vi "Record Defaults in Log File.vi"(6 "Application":refnum<class "Application.lvclass">, 7 "Position":u32, 8 "error in (no error)":errorcluster, 11 "Parameter Loader in":refnum<class "Parameter Loader.lvclass">) -> (0 "error out":errorcluster)   [LabVIEW 2015, in "Load Defaults.lvclass"]
uses:
  Load Defaults.lvclass
  Classes/Parameter Loader/Class/Parameter Loader.lvclass
  Classes/Application/Class/Application.lvclass
  <vilib>/Cree, Inc/Cree Test Framework/Core Launcher/Core Manager Methods -- Enum.ctl
  <vilib>/Cree, Inc/Cree Test Framework/Core Launcher/Core Launcher.lvlib
  <vilib>/Cree, Inc/Cree Test Framework/Classes/Data/Data Repo/Class/Data Repo.lvclass
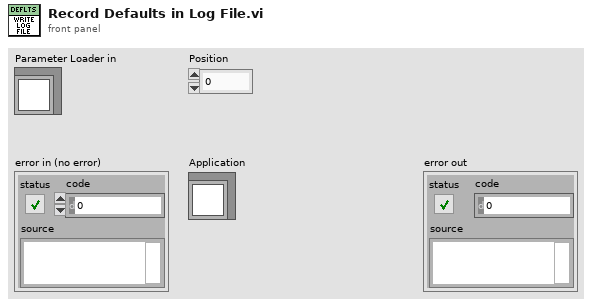
[diagram p1: front panel]
types:
  T1 = typedef "Core Launcher.lvlib/Core Manager Methods -- Enum.ctl" = enum16{"Spawn Objects", "Get Objects", "Destroy Objects"}
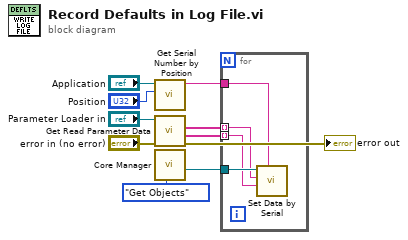
[diagram p0: block diagram]
diagram:
  n1 = call "Get Serial Number by Position.vi"("Position"="Position", "Application.lvclass"="Application") -> ("Value"=w1:string)  [unwired: 9 in]
  n2 = call "Get Read Parameter Data.vi"("error in (no error)"="error in (no error)", "Parameter Loader in"="Parameter Loader in") -> ("error out"=→"error out":errorcluster, "Parameter Data"=w7:string[], "Parameter Headers"=w8:string[])  [unwired: 6 in, 1 out]
  n3 = call <vilib>:"Core Manager.vi"("Method"=Core_Manager_Methods_--_Enum."Get Objects") -> ("Data Repo"=w6:refnum<class "Data Repo.lvclass">)  [unwired: 6 in, 4 out]
  n4 = for {
    tunnel: w8 -> [w12] mode=indexing
    tunnel: w7 -> [w11] mode=indexing
    tunnel: w6 -> [w13]
    tunnel: w1 -> [w14]
    n5 = call <vilib>:"Set Data by Serial.vi"("Serial"=w14, "Value"=w11, "Header"=w12, "Acrobat Template in"=w13) -> ()  [unwired: 6 in, 2 out]
  }
